vi "normalize_arrau.vi"(11 "Array in":i16[](array[numeric])) -> (3 "Array out":dbl[](array[numeric]))   [LabVIEW 2011]
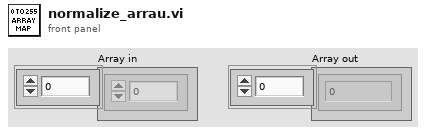
[diagram p1: front panel]
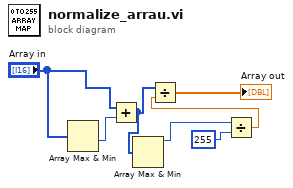
[diagram p0: block diagram]
diagram:
  n1 = Array Max & Min(array="Array in") -> (min value=w3:i16)  [unwired: 3 out]
  n2 = Add(x="Array in", y=w3) -> (x+y=w2:i16[])
  n3 = Array Max & Min(array=w2) -> (max value=w1:i16)  [unwired: 3 out]
  n4 = Divide(x=w1, y=i16 255) -> (x/y=w6:dbl)
  n5 = Divide(x=w2, y=w6) -> (x/y=→"Array out":dbl[])
